vi "Configure LPC.vi"(0 "VISA resource name":refnum<visa-resource-name>="GPIB0::3::INSTR", 1 "power":dbl[unit]=0.005, 5 "wavelength":dbl[unit]=8.300000000000001e-07, 7 "Transmission":dbl=50.0, 9 "control mode":T1(ring), 11 "error in (no error)":errorcluster, 12 "front-panel controls":enum16{"enabled", "disabled"}(ring)) -> (4 "VISA resource name out":refnum<visa-resource-name>, 15 "error out":errorcluster)   [LabVIEW 2009, in "BEOC LPC.lvlib"]
doc: "Configures the most important (to us) settings for the LPC (laser power controller)."
uses:
  BEOC LPC.lvlib
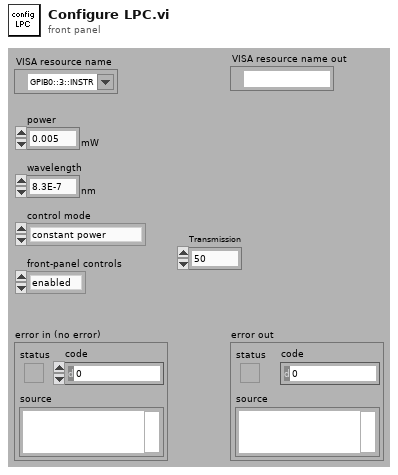
[diagram p1: front panel]
types:
  T1 = enum16{"constant power", "constant transmission"}
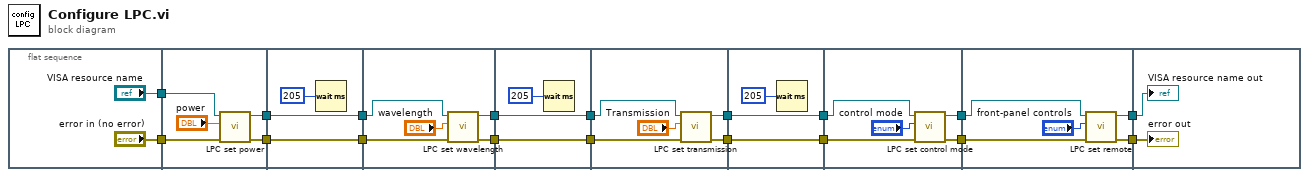
[diagram p0: block diagram]
diagram:
  n1 = flat-sequence {
    tunnel: ["VISA resource name"] -> w18
    tunnel: ["error in (no error)"] -> w17
    tunnel: w18 -> [w24]
    tunnel: w17 -> [w23]
    tunnel: [w22] -> w12
    tunnel: [w21] -> w10
    tunnel: w12 -> [w28]
    tunnel: [w28] -> w11
    tunnel: w10 -> [w27]
    tunnel: [w27] -> w9
    tunnel: w11 -> [w32]
    tunnel: w9 -> [w31]
    tunnel: [w30] -> w8
    tunnel: [w29] -> w7
    tunnel: w8 -> [w36]
    tunnel: [w36] -> w6
    tunnel: w7 -> [w35]
    tunnel: [w35] -> w5
    tunnel: w6 -> [w41]
    tunnel: [w40] -> w4
    tunnel: w5 -> [w38]
    tunnel: [w39] -> w2
    tunnel: w4 -> [w44]
    tunnel: [w44] -> w3
    tunnel: w2 -> [w43]
    tunnel: [w43] -> w1
    tunnel: w3 -> [w48]
    tunnel: w1 -> [w47]
    tunnel: [w46] -> w16
    tunnel: [w45] -> w15
    tunnel: w16 -> [w53]
    tunnel: w15 -> [w52]
    tunnel: [w51] -> w14
    tunnel: [w50] -> w13
    tunnel: w14 -> [w56]
    tunnel: w13 -> [w55]
    frame #0 {
    }
    frame #1 {
      n2 = call "LPC set power.vi"("error in (no error)"=w23, "power"="power", "VISA resource name"=w24) -> ("error out"=w21:errorcluster, "VISA resource name out"=w22:refnum<visa-resource-name>)  [unwired: 7 out]
    }
    frame #2 {
      n3 = Wait (ms)(milliseconds to wait=u32 205) -> ()  [unwired: 1 out]
    }
    frame #3 {
      n4 = call "LPC set wavelength.vi"("error in (no error)"=w31, "wavelength"="wavelength", "VISA resource name"=w32) -> ("error out"=w29:errorcluster, "VISA resource name out"=w30:refnum<visa-resource-name>)  [unwired: 7 out]
    }
    frame #4 {
      n5 = Wait (ms)(milliseconds to wait=u32 205) -> ()  [unwired: 1 out]
    }
    frame #5 {
      n6 = call "LPC set transmission.vi"("error in (no error)"=w38, "transmission (%)"="Transmission", "VISA resource name"=w41) -> ("error out"=w39:errorcluster, "VISA resource name out"=w40:refnum<visa-resource-name>)  [unwired: 7 in]
    }
    frame #6 {
      n7 = Wait (ms)(milliseconds to wait=u32 205) -> ()  [unwired: 1 out]
    }
    frame #7 {
      n8 = call "LPC set control mode.vi"("error in (no error)"=w47, "control mode"="control mode", "VISA resource name"=w48) -> ("error out"=w45:errorcluster, "VISA resource name out"=w46:refnum<visa-resource-name>)  [unwired: 7 out]
    }
    frame #8 {
      n9 = call "LPC set remote.vi"("error in (no error)"=w52, "front-panel controls"="front-panel controls", "VISA resource name"=w53) -> ("error out"=w50:errorcluster, "VISA resource name out"=w51:refnum<visa-resource-name>)  [unwired: 7 out]
    }
    frame #9 {
      "VISA resource name out" <- w56
      "error out" <- w55
    }
  }
